vi "Decimate 2D By Percentage.vi"(6 "Width":u32, 8 "error in (no error)":errorcluster, 9 "Xmin [%]":dbl, 10 "Xmax [%]":dbl, 11 "Data to Decimate":dbl[][](array[numeric])) -> (0 "error out":errorcluster, 3 "Decimated Data":dbl[][](array[numeric]))   [LabVIEW 2022 SP3, in "Decimation.lvlib"]
doc: "Decimate 2D array to optimize the density of points per pixel to 2 : Min & Max per pixel."
uses:
  Decimation.lvlib
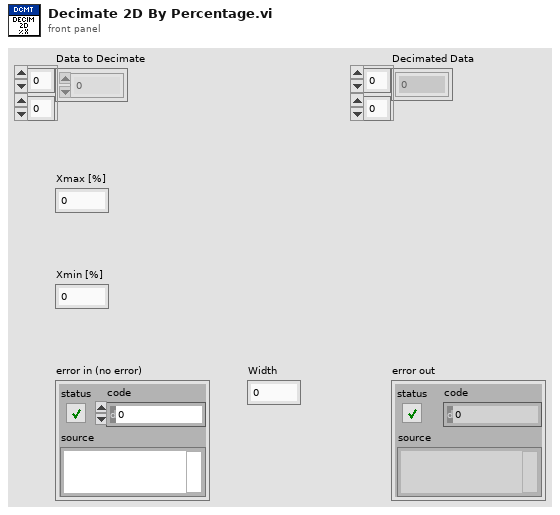
[diagram p1: front panel]
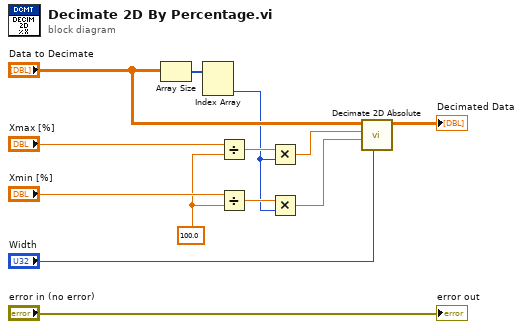
[diagram p0: block diagram]
diagram:
  w8 = 100.0 ("y")
  n1 = Array Size(array="Data to Decimate") -> (size(s)=w5:i32[])
  n2 = Index Array(array=w5) -> (element #2=w4:i32)  [unwired: 2 in, 1 out]
  n3 = Divide(x="Xmax [%]", y=w8) -> (x/y=w6:dbl)
  n4 = Divide(x="Xmin [%]", y=w8) -> (x/y=w7:dbl)
  n5 = Multiply(x=w6, y=w4) -> (x*y=w2:dbl)
  n6 = Multiply(x=w7, y=w4) -> (x*y=w3:dbl)
  n7 = call "Decimate 2D Absolute.vi"("Width"="Width", "Xmin"=w3, "Xmax"=w2, "Data to Decimate"="Data to Decimate") -> ("Decimated Data"=→"Decimated Data":dbl[][])  [unwired: 6 in, 1 out]
  "error out" <- "error in (no error)"
